vi "cook.vi"(8 "error in (no error)":errorcluster, 11 "Broil in":refnum<class "Broil.lvclass">) -> (0 "error out":errorcluster, 3 "Broil out":refnum<class "Broil.lvclass">)   [LabVIEW 2010, in "CookBehaviors.lvlib" / "Broil.lvclass"]
uses:
  Broil.lvclass
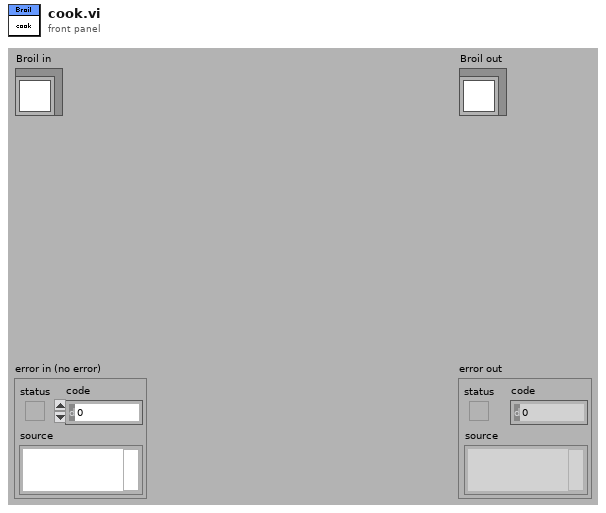
[diagram p1: front panel]
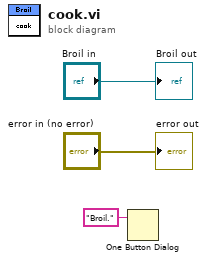
[diagram p0: block diagram]
diagram:
  n1 = One Button Dialog(message="Broil.") -> ()  [unwired: 1 in, 1 out]
  "error out" <- "error in (no error)"
  "Broil out" <- "Broil in"
